vi "GetMessageLength.vi"(8 "error in (no error)":errorcluster, 11 "TCP_Server_Connection_Handler in":refnum<class "TCP_Server_Connection_Handler.lvclass">) -> (0 "error out":errorcluster, 3 "TCP_Server_Connection_Handler out":refnum<class "TCP_Server_Connection_Handler.lvclass">)   [LabVIEW 2023, in "TCP_Server_Connection_Handler.lvlib" / "TCP_Server_Connection_Handler.lvclass"]
uses:
  TCP_Server_Connection_Handler.lvclass
  TCP_Server_Connection_Handler.lvclass/TCP_Server_Connection_Handler.ctl
  <vilib>/ActorFramework/Actor/Actor.lvclass
  <vilib>/ActorFramework/Stop Msg/Stop Msg.lvclass
  TCP_Server_Connection_Handler Messages/GetMessage Msg/GetMessage Msg.lvclass
  TCP_Server_Connection_Handler Messages/FindMessageStart Msg/FindMessageStart Msg.lvclass
  TCP_Server_Connection_Handler Messages/Increment Bytes Received Msg/Increment Bytes Received Msg.lvclass
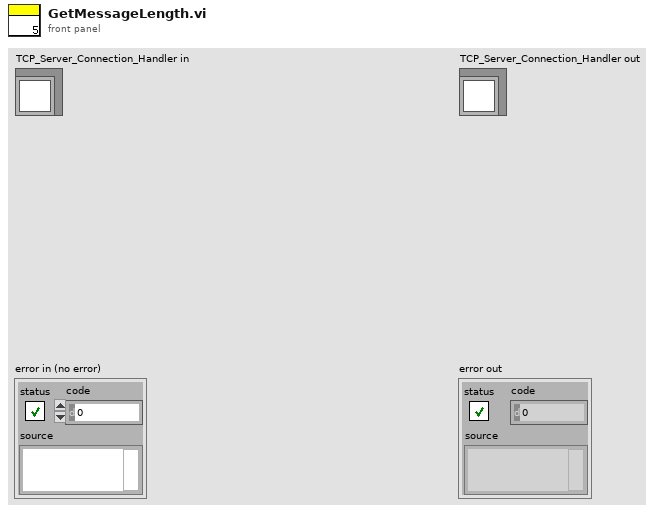
[diagram p1: front panel]
types:
  T1 = typedef "TCP_Listener.lvlib/ConnectionInformation.ctl" = cluster{"Connection number":i32, "Remote Address":string, "Remote Port":u16, "Connection ID":refnum<k5>, "bytes received":i32, "bytes  sent":i32}
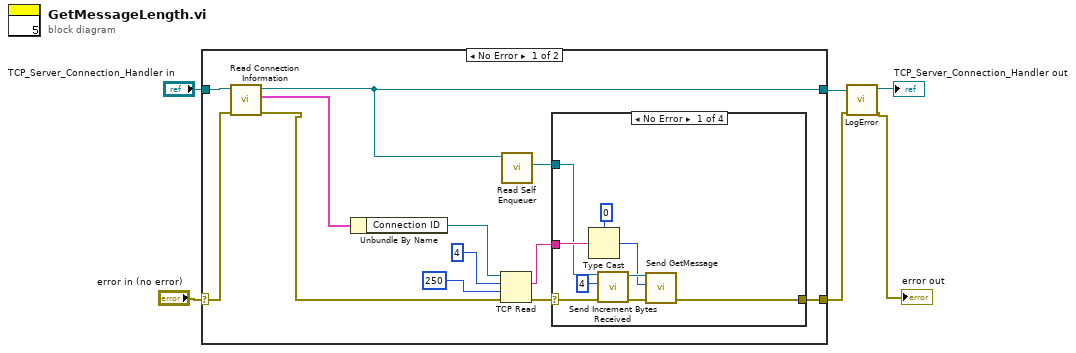
[diagram p0: block diagram]
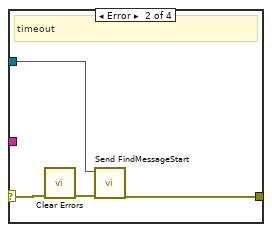
[diagram p2: hidden frame]
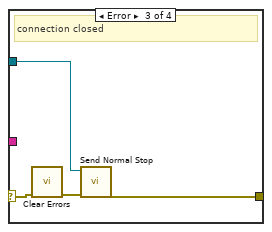
[diagram p3: hidden frame]
diagram:
  n1 = case shown="No Error" "error in (no error)" {
    selector: "error in (no error)" -> [w12 w38]
    tunnel: [w8 w38] -> w2
    tunnel: [w7 w37] -> w4
    tunnel: "TCP_Server_Connection_Handler in" -> [w13 w37]
    frame No Error {
      n2 = call "Read Connection Information.vi"("error in (no error)"=w12, "TCP_Server_Connection_Handler in"=w13) -> ("error out"=w14:errorcluster, "Connection Information"=w18:T1, "TCP_Server_Connection_Handler out"=w7:refnum<class "TCP_Server_Connection_Handler.lvclass">)  [unwired: 7 in]
      n3 = Unbundle By Name(w18) -> ("Connection ID"=w17:refnum<k5>)
      n4 = TCP Read(connection ID=w17, bytes to read=4, error in (no error)=w14, 9:250 ("timeout ms (25000)")) -> (data out=w15:string, error out=w10:errorcluster)  [unwired: 1 in, 1 out]
      n5 = call <vilib>:"Read Self Enqueuer.vi"("Actor"=w7) -> ("Self Enqueuer"=w9:refnum<class "Message Enqueuer.lvclass">)  [unwired: 10 in]
      n6 = case shown="No Error" w10 {
        selector: w10 -> [w24 w31 w33 w36]
        tunnel: w15 -> [w27 _ _ _]
        tunnel: w9 -> [w22 w30 w35 _]
        tunnel: [w25 w28 w34 w36] -> w8
        frame No Error {
          n7 = Type Cast(type=0, x=w27) -> (*(type *) &x=w19:i32)
          n8 = call "Send Increment Bytes Received.vi"("error in (no error)"=w24, "Increment"=4, "Message Enqueuer"=w22) -> ("error out"=w23:errorcluster, "Message Enqueuer out"=w20:refnum<class "Message Enqueuer.lvclass">)  [unwired: 7 in]
          n9 = call "Send GetMessage.vi"("error in (no error)"=w23, "Message length"=w19, "Message Enqueuer"=w20) -> ("error out"=w25:errorcluster)  [unwired: 7 in, 1 out]
        }
        frame Error {
          # "timeout"
          n10 = call <vilib>:"Clear Errors.vi"("error in (no error)"=w31) -> ("error out"=w29:errorcluster)  [unwired: 5 in, 1 out]
          n11 = call "Send FindMessageStart.vi"("error in (no error)"=w29, "Message Enqueuer"=w30) -> ("error out"=w28:errorcluster)  [unwired: 8 in, 1 out]
        }
        frame Error {
          # "connection closed"
          n12 = call <vilib>:"Clear Errors.vi"("error in (no error)"=w33) -> ("error out"=w32:errorcluster)  [unwired: 5 in, 1 out]
          n13 = call <vilib>:"Send Normal Stop.vi"("error in (no error)"=w32, "Message Enqueuer"=w35) -> ("error out"=w34:errorcluster)  [unwired: 9 in]
        }
        frame Default {
        }
      }
    }
    frame Error {
    }
  }
  n14 = call "LogError.vi"("error in (no error)"=w2, "TCP_Server_Connection_Handler in"=w4) -> ("error out"=→"error out":errorcluster, "TCP_Server_Connection_Handler out"=→"TCP_Server_Connection_Handler out":refnum<class "TCP_Server_Connection_Handler.lvclass">)  [unwired: 8 in]
